vi "SysDef.CreateChannel.vi"(7 "GUID":string="03D3BB99-1485-13A6-561D1F898F032919" caption="GUID (Default Channel)", 8 "error in (no error)":errorcluster, 9 "Channel":T1, 10 "Name":string, 11 "nodeID":u64) -> (0 "error out":errorcluster, 1 "New NodeID":u64, 2 "newItem":bool, 3 "nodeID out":u64)   [LabVIEW 2024, in "Advanced System Definition.lvlib"]
uses:
  Advanced System Definition.lvlib
  C:/NetCore/niveristand-custom-device-development-tools/advanced-sysdef-api/Source/SysDef API/SysDef.CreateChannel.vi/NationalInstruments.VeriStand.SystemDefinitionAPI
  NationalInstruments.VeriStand.SystemDefinitionAPI
  <vilib>/NI VeriStand/Custom Device API/Custom Device API.lvlib
  <vilib>/NI VeriStand/Custom Device API/Custom Device Channel Type.ctl
  <vilib>/NI VeriStand/Custom Device API/Custom Device Channel.ctl
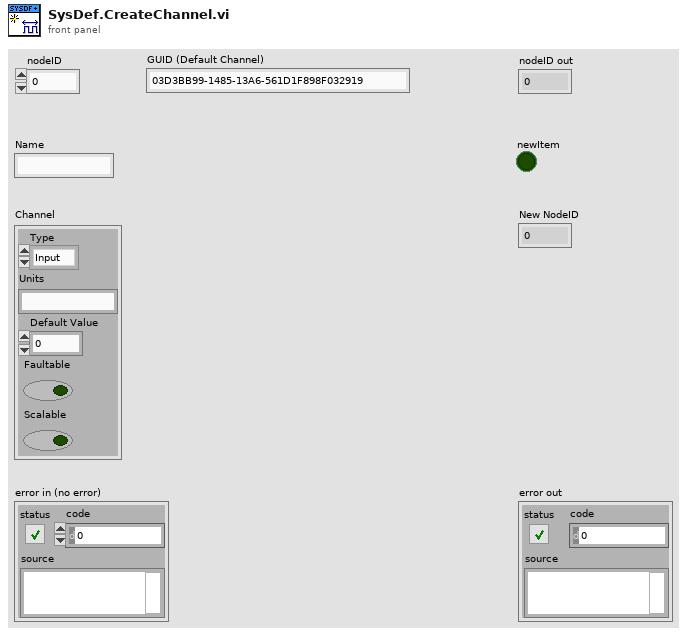
[diagram p1: front panel]
types:
  T1 = typedef "Custom Device API.lvlib/Custom Device Channel.ctl" = cluster{"Type":T2, "Units":string, "Default Value":dbl, "Faultable":bool, "Scalable":bool}
  T2 = typedef "Custom Device API.lvlib/Custom Device Channel Type.ctl" = enum16{"Input", "Output"}
  T3 = typedef "Custom Device API.lvlib/Custom Device Item Ref.ctl" = u64
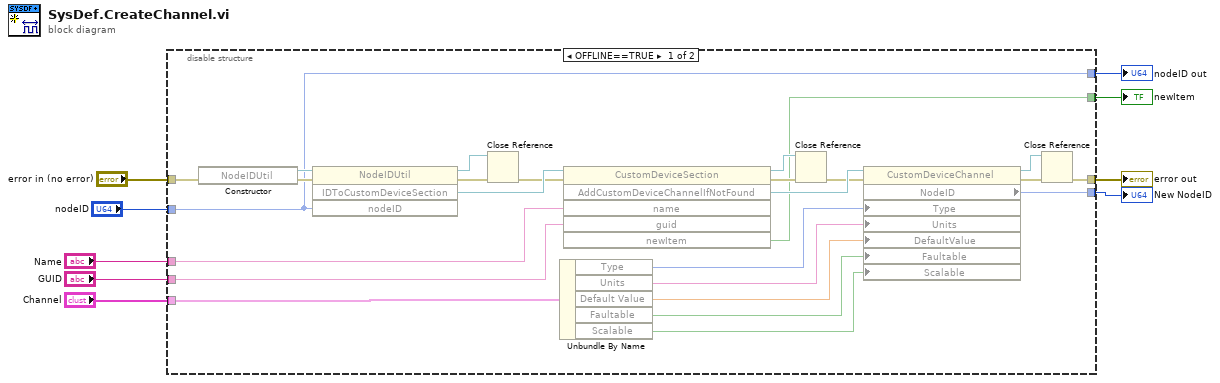
[diagram p0: block diagram]
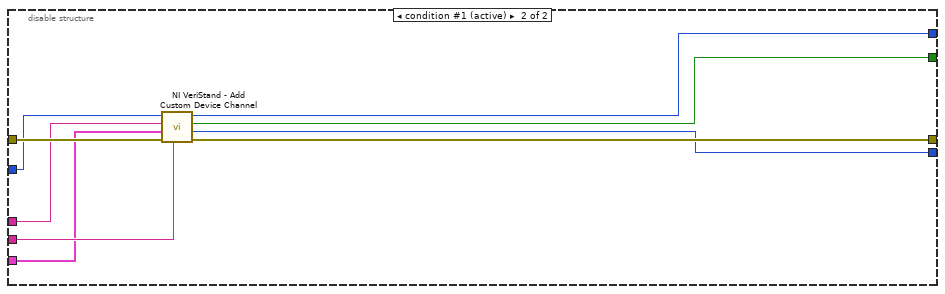
[diagram p2: hidden frame]
diagram:
  n1 = disable-structure shown="OFFLINE==TRUE" {
    disable-tunnel: "nodeID" -> [w10 w42]
    disable-tunnel: "error in (no error)" -> [w31 w43]
    disable-tunnel: [w29 w36] -> w8
    disable-tunnel: [w15 w37] -> w7
    disable-tunnel: "Name" -> [w14 w40]
    disable-tunnel: "GUID" -> [w13 w41]
    disable-tunnel: "Channel" -> [w12 w39]
    disable-tunnel: [w11 w38] -> w3
    disable-tunnel: [w10 w35] -> w1
    frame condition #0 {
      n2 = constructor class="NodeIDUtil"(error in=w31) -> (reference out=w33:refnum<k24>, error out=w32:errorcluster)  [unwired: 2 in, 1 out]
      n3 = invoke class="NodeIDUtil" method="IDToCustomDeviceSection"(reference=w33, error in=w32, "nodeID"=w10) -> (reference out=w30:refnum<k24>, error out=w17:errorcluster, "IDToCustomDeviceSection"=w34:refnum<k24>)  [unwired: 1 in, 1 out]
      n4 = Close Reference(reference=w30, error in (no error)=w17) -> (error out=w16:errorcluster)
      n5 = Unbundle By Name(w12) -> ("Type"=w20:T2, "Units"=w24:string, "Default Value"=w23:dbl, "Faultable"=w22:bool, "Scalable"=w21:bool)
      n6 = invoke class="CustomDeviceSection" method="AddCustomDeviceChannelIfNotFound"(reference=w34, error in=w16, "name"=w14, "guid"=w13) -> (reference out=w27:refnum<k24>, error out=w28:errorcluster, "AddCustomDeviceChannelIfNotFound"=w26:refnum<k24>, "newItem"=w11:bool)  [unwired: 2 in, 2 out]
      n7 = Close Reference(reference=w27, error in (no error)=w28) -> (error out=w25:errorcluster)
      n8 = property class="CustomDeviceChannel"(reference=w26, error in=w25, "Type"=w20, "Units"=w24, "DefaultValue"=w23, "Faultable"=w22, "Scalable"=w21) -> (reference out=w19:refnum<k24>, error out=w18:errorcluster, "NodeID"=w29:u64)
      n9 = Close Reference(reference=w19, error in (no error)=w18) -> (error out=w15:errorcluster)
    }
    frame condition #1 (active) {
      n10 = call <vilib>:"NI VeriStand - Add Custom Device Channel.vi"("GUID (Default Channel)"=w41, "error in (no error)"=w43, "Channel"=w39, "Channel Name"=w40, "Parent Ref in"=w42) -> ("error out"=w37:errorcluster, "Channel Ref"=w36:T3, "Newly Created?"=w38:bool, "Parent Ref out"=w35:T3)  [unwired: 3 in]
    }
  }
  "New NodeID" <- w8
  "nodeID out" <- w1
  "error out" <- w7
  "newItem" <- w3
